vi "Toggle Filter Enabled State.vi"(4 "Click Coordinates":T1, 6 "MulticolumnListbox in":refnum<vi>, 7 "Caller Enqueuer":refnum<class "Message Enqueuer.lvclass">, 8 "error in":errorcluster, 10 "Filter Array in":variant[](array[variant])) -> (0 "error out":errorcluster, 2 "Filter Array out":variant[](array[variant]))   [LabVIEW 2018, in "Assert API Components.lvlib" / "Assert Display.lvlib" / "Filter Config Display.lvlib" / "Filter Config Display.lvclass"]
uses:
  Filter Config Display.lvclass
  <vilib>/Utility/miscctls.llb/LVPoint32TypeDef.ctl
  <vilib>/ActorFramework/Message Enqueuer/Message Enqueuer.lvclass
  Assert API Components/Filter Configurations/Base Filter.lvclass
  Assert Display/Components/Item Configuration.ctl
  Assert Display/Components/Item Type.ctl
  Assert API Components/Filter Configurations/Base Filter.lvclass/Base Filter.ctl
  Assert Display/Assert Display Messages/Remove Item Msg/Remove Item Msg.lvclass/Remove Item Msg.ctl
  <vilib>/ActorFramework/Message Enqueuer/Message Enqueuer.lvclass/Message Enqueuer.ctl
  Assert Display/Assert Display Messages/New Item Msg/New Item Msg.lvclass/New Item Msg.ctl
  <vilib>/ActorFramework/Message Enqueuer/Enqueue.vi
  Assert Display/Assert Display Messages/Remove Item Msg/Remove Item Msg.lvclass
  C:/Program Files (x86)/National Instruments/LabVIEW 2018/vi.lib/ActorFramework/Message/Message.lvclass
  Assert Display/Assert Display Messages/New Item Msg/New Item Msg.lvclass
  <vilib>/Utility/LVClass/Get LV Class Name.vi
  <resource>/AFDebug/Generate Trace for Message.vi
  <vilib>/ActorFramework/Message Priority Queue/Priority Enqueue.vi
  Assert Display/Assert Display/Assert Display.lvclass
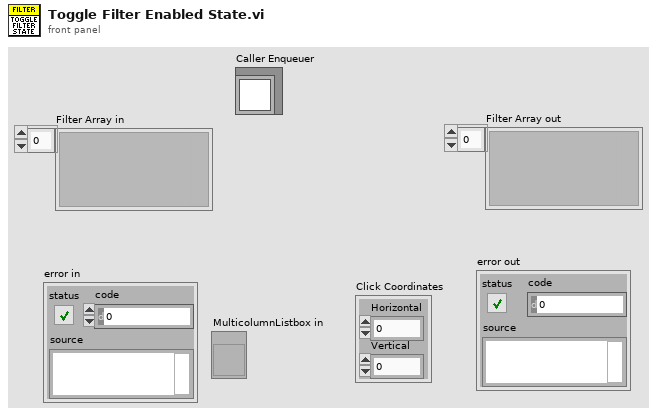
[diagram p1: front panel]
types:
  T1 = typedef "LVPoint32TypeDef.ctl" = cluster{"Horizontal":i32, "Vertical":i32}
  T2 = typedef "LVRowAndColumnTypeDef.ctl" = cluster{"Row":i32, "Column":i32}
  T3 = typedef "Assert API Components.lvlib/Assert Display.lvlib/Assert Display.lvclass/Item Type.ctl" = enum16{"Filter"}
  T4 = typedef "Assert API Components.lvlib/Assert Display.lvlib/Assert Display.lvclass/Item Configuration.ctl" = cluster{"Item Type":T3, "Configuration":variant}
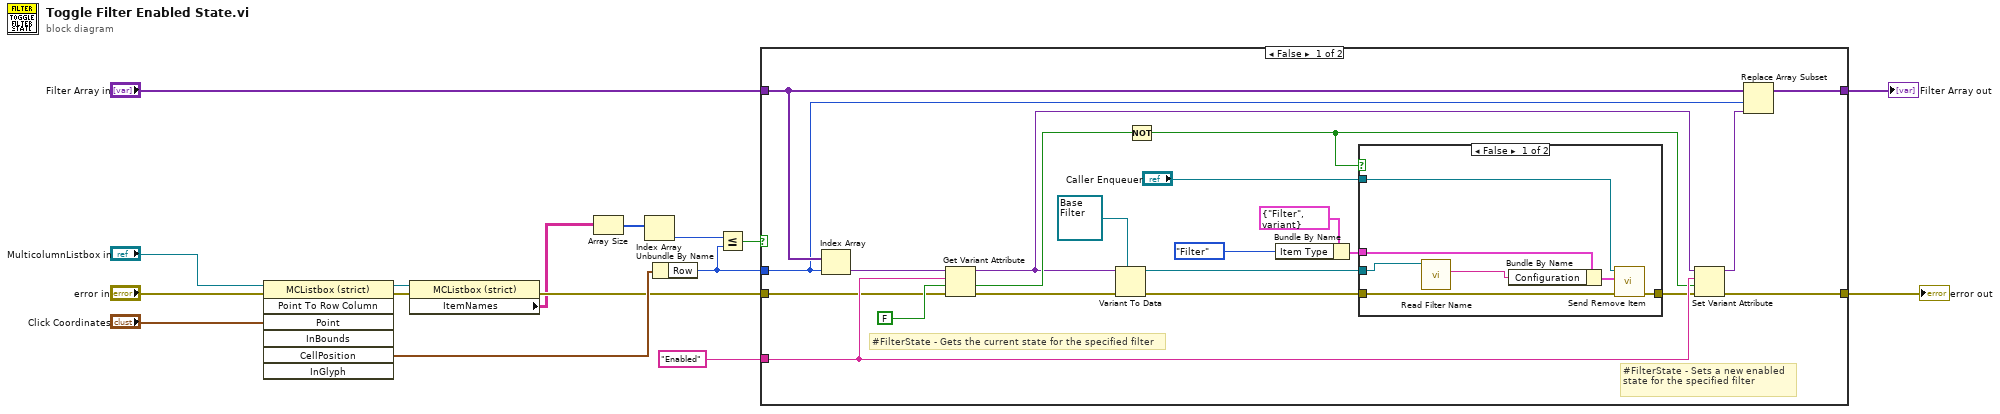
[diagram p0: block diagram]
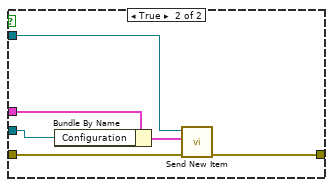
[diagram p2: hidden frame]
diagram:
  n1 = invoke on="Invoke Node" class="MCListbox (strict)" method="Point To Row Column"(reference="MulticolumnListbox in", error in="error in", "Point"="Click Coordinates") -> (reference out=w6:refnum<vi>, error out=w8:errorcluster, "CellPosition"=w16:T2)  [unwired: 4 in, 4 out]
  n2 = property class="MCListbox (strict)"(reference=w6, error in=w8) -> (error out=w7:errorcluster, "ItemNames"=w5:string[][])  [unwired: 1 out]
  n3 = Array Size(array=w5) -> (size(s)=w4:i32[])
  n4 = Index Array(array=w4) -> (element=w2:i32)  [unwired: 1 in]
  n5 = Unbundle By Name(w16) -> ("Row"=w3:i32)
  n6 = Less Or Equal?(x=w2, y=w3) -> (x <= y?=w1:bool)
  n7 = case shown="False" w1 {
    tunnel: "Enabled" ("name") -> [w25 _]
    tunnel: "Filter Array in" -> [w23 w51]
    tunnel: [w21 w52] -> w11
    tunnel: [w20 w51] -> w10
    tunnel: w7 -> [w18 w52]
    tunnel: w3 -> [w17 _]
    frame False {
      # "#FilterState - Sets a new enabled state for the specified filter"
      # "#FilterState - Gets the current state for the specified filter"
      n8 = Index Array(array=w23, index=w17) -> (element=w37:variant)
      n9 = Get Variant Attribute(Variant=w37, name=w25, default value (empty Variant)=FALSE, error in=w18) -> (duplicate Variant=w27:variant, value=w35:bool, error out=w26:errorcluster)  [unwired: 1 out]
      n10 = Variant To Data(error in=w26, type=refnum<class "Base Filter.lvclass"> refnum ("Assert API Components.lvlib:Base Filter.lvclass"), Variant=w27) -> (data=w29:refnum<class "Base Filter.lvclass">, error out=w28:errorcluster)
      n11 = Not(x=w35) -> (.not. x?=w24:bool)
      n12 = Bundle By Name(cluster=T4 {"Item Type"=enum."Filter", "Configuration"=variant} ("Item Configuration"), "Item Type"=Item_Type."Filter") -> (w30:T4)
      n13 = case shown="False" w24 {
        tunnel: "Caller Enqueuer" -> [w44 w50]
        tunnel: w30 -> [w43 w49]
        tunnel: w29 -> [w42 w48]
        tunnel: w28 -> [w40 w46]
        tunnel: [w39 w45] -> w19
        frame False {
          n14 = call "Read Filter Name.vi"("Base Filter in"=w42) -> ("Filter Name"=w41:string)  [unwired: 10 in]
          n15 = Bundle By Name(cluster=w43, "Configuration"=w41) -> (w38:T4)
          n16 = call "Send Remove Item.vi"("error in (no error)"=w40, "Item Configuration"=w38, "Message Enqueuer"=w44) -> ("error out"=w39:errorcluster)  [unwired: 7 in, 1 out]
        }
        frame True {
          n17 = Bundle By Name(cluster=w49, "Configuration"=w48) -> (w47:T4)
          n18 = call "Send New Item.vi"("error in (no error)"=w46, "Item Configuration"=w47, "Message Enqueuer"=w50) -> ("error out"=w45:errorcluster)  [unwired: 7 in, 1 out]
        }
      }
      n19 = Set Variant Attribute(Variant=w27, name=w25, value=w24, error in=w19) -> (Variant out=w22:variant, error out=w21:errorcluster)  [unwired: 1 out]
      n20 = Replace Array Subset(array=w23, new element=w22, index=w17) -> (w20:variant[])
    }
    frame True {
    }
  }
  "Filter Array out" <- w10
  "error out" <- w11
